vi "AxesPositions.vi"(0 "System no.":i32=1 min=1 step=1, 5 "error in":errorcluster) -> (19 "error out":errorcluster)   [LabVIEW 2014]
doc: "This VI allows to save position information to a text file. Also the position information from a text file can be opened again.\nPressing on the \"Stop Motion (F10)\" or the F10 key will send a \"#24\" command to the controller to stop the motion of every axis.\nThis VI opens modal so that the communication, especially the STOP command, is not disturbed by any other processes."
uses:
  C:/ProgramData/PI/LabVIEW/Low Level/General command.llb/Global2 (Array).vi
panel:
  in  "Move to target":bool[](array[boolean])
  in  "Save to file":bool
  in  "Load from file":bool
  in  "Current to Target":bool
  in  "Target Position":dbl[](array[numeric]) format="%.6f"
  out "Conn. axes":string[](array[string])
  out "Current Position":dbl[](array[numeric]) format="%.6f"
  in  "Stop Motion":bool
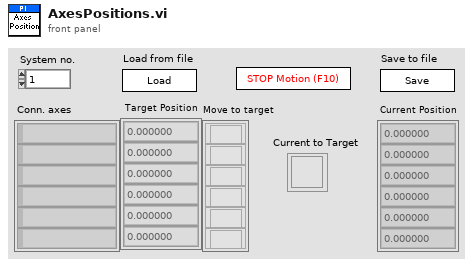
[diagram p1: front panel]
types:
  T1 = enum16{"open", "replace", "create", "open or create", "replace or create", "replace or create with confirmation"}
  T2 = typedef "Controller names.ctl" = enum16{"None", "Analog", "C-702", "C-413", "C-414", "C-843", "C-843.PM", "C-844", "C-848", "C-865", "C-866", "C-867", "C-877", "C-880", "C-884", "C-885", "C-886", "C-887", "C-891", "E-135", "E-516", "E-517", "E-518", "E-709", "E-710", "E-712", "E-725", "E-727", "E-753", "E-754", "E-755", "E-761", "E-816", "E-861", "E-870", "E-871", "E-872", "E-873", "E-874", "F-206", "HydraPollux", "M-840", "M-850", "M-8X0", "Mercury", "Mercury_GCS", "PI_GCS2"}
  T3 = cluster{"Conn. axes":string[], "Controller name":T2}[]
  T4 = cluster{"Conn. axes":string[], "Controller name":T2}
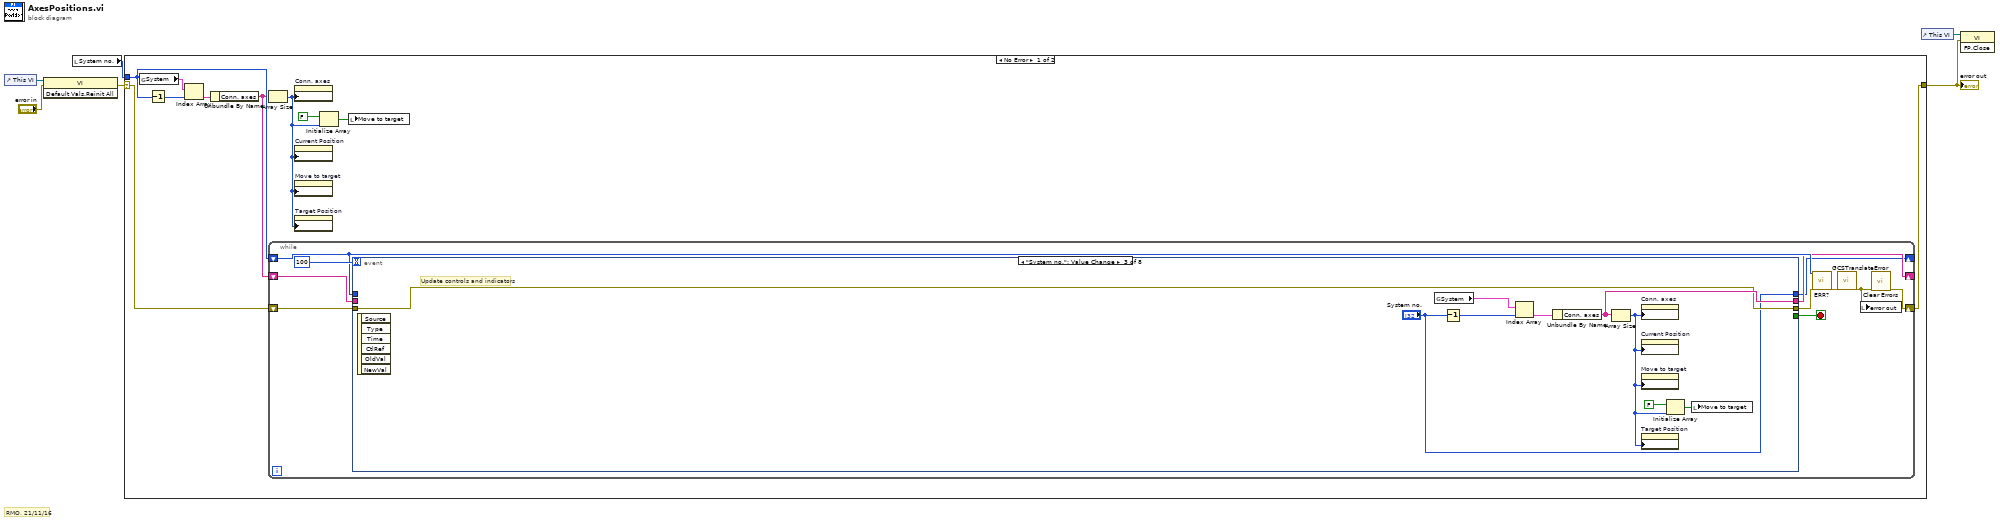
[diagram p0: block diagram]
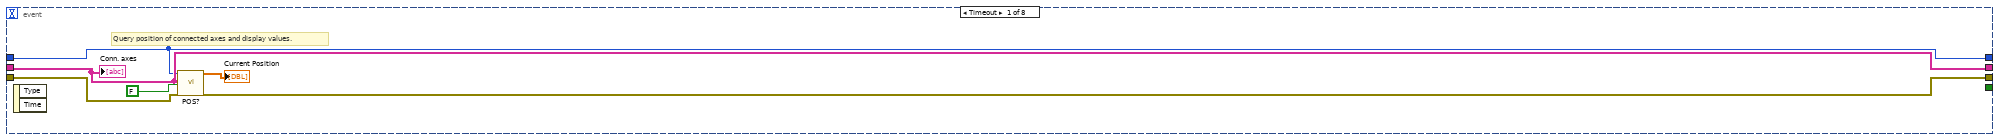
[diagram p2: hidden frame]
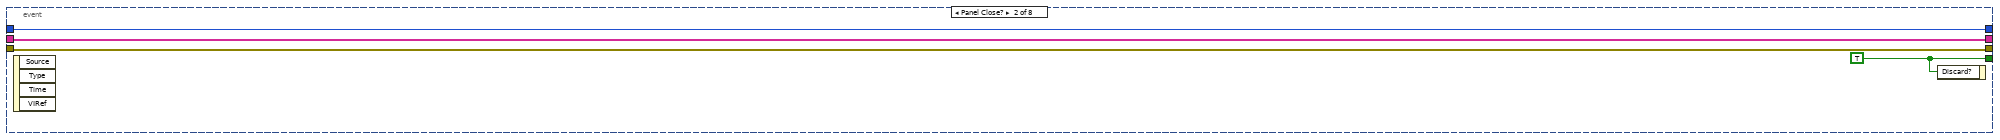
[diagram p3: hidden frame]
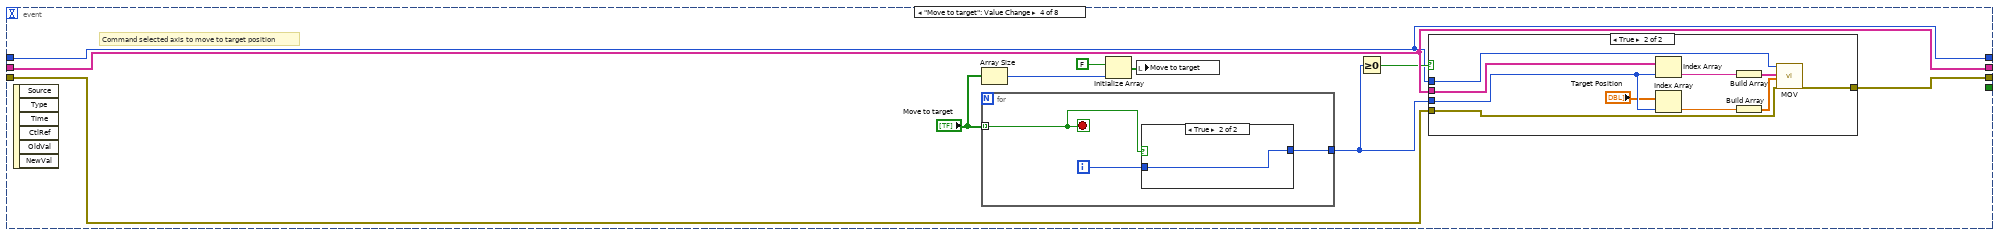
[diagram p4: hidden frame]
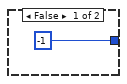
[diagram p6: hidden frame]
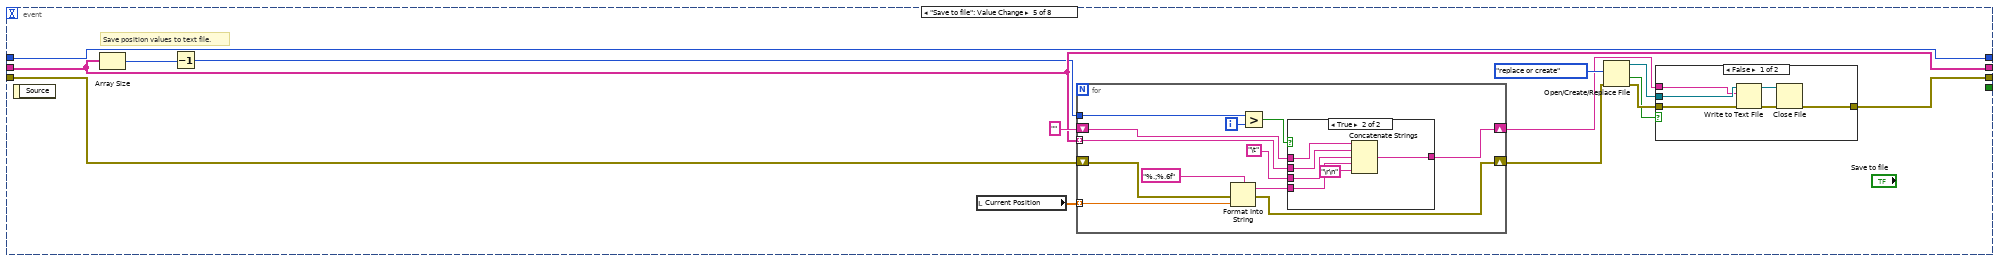
[diagram p7: hidden frame]
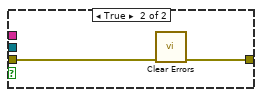
[diagram p8: hidden frame]
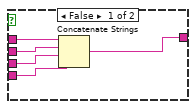
[diagram p9: hidden frame]
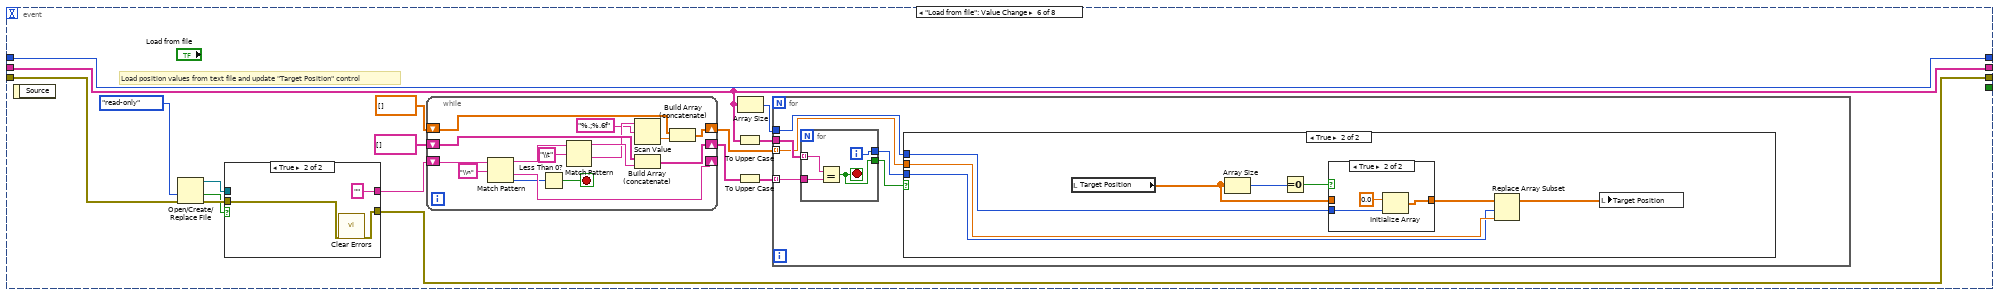
[diagram p10: hidden frame]
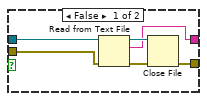
[diagram p11: hidden frame]
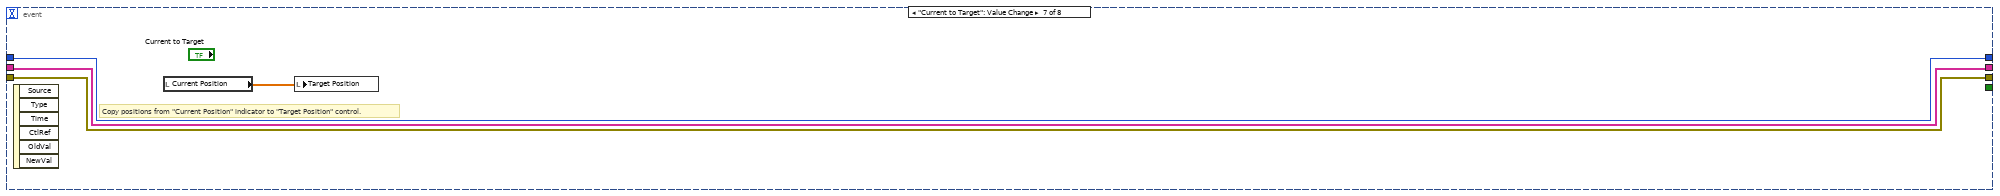
[diagram p14: hidden frame]
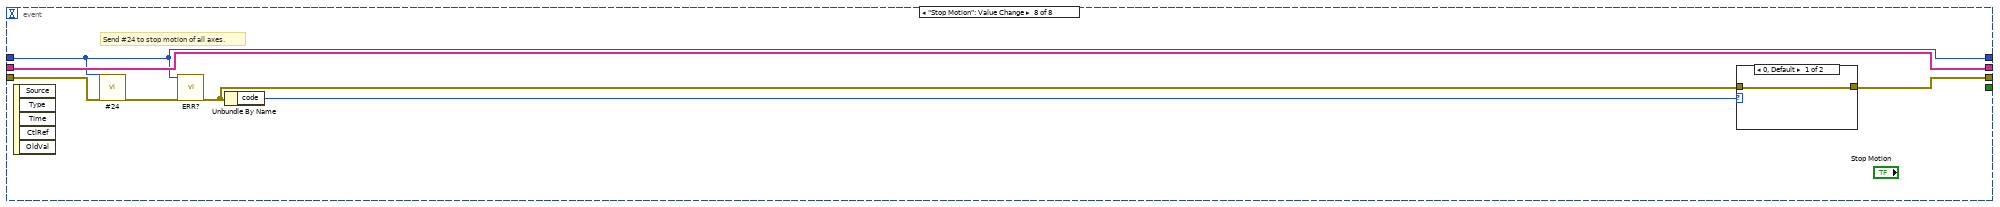
[diagram p15: hidden frame]
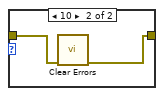
[diagram p16: hidden frame]
diagram:
  # "RMO, 21/11/16"
  n1 = control-ref of="This VI"() -> (w5:refnum<vi>)
  n2 = invoke class="VI" method="Default Vals.Reinit All"(reference=w5, error in="error in") -> (error out=w3:errorcluster)  [unwired: 1 in, 2 out]
  n3 = local read "System no."() -> (w1:i32)
  n4 = case shown="No Error" w3 {
    selector: w3 -> [w11 w194]
    tunnel: [w13 w194] -> w6
    tunnel: w1 -> [w12 _]
    frame No Error {
      n5 = global read "Global2 (Array).vi" "System"() -> (w16:T3)
      n6 = Decrement(x=w12) -> (x-1=w15:i32)
      n7 = Index Array(array=w16, index=w15) -> (element=w14:T4)
      n8 = Unbundle By Name(w14) -> ("Conn. axes"=w10:string[])
      n9 = Array Size(array=w10) -> (size(s)=w7:i32)
      n10 = while {
        shift-right: [w20] -> w13
        shift-left: w11 -> [w26]
        shift-right: [w18] -> _
        shift-left: w10 -> [w27]
        shift-right: [w17] -> _
        shift-left: w12 -> [w21]
        stop <- w25 stop-if-true
        n11 = event shown="[2] \"System no.\": Value Change" {
          selector: _ -> [_ _ _ _ _ _ _ _]
          dyn-events: _ -> [_ _ _ _ _ _ _ _]
          timeout: 100 -> [_ _ _ _ _ _ _ _]
          tunnel: w27 -> [w29 w36 _ w52 w84 w120 w181 w190]
          tunnel: w26 -> [w33 w35 w39 w49 w81 w133 w183 w189]
          tunnel: [w32 w35 w39 w48 w75 w122 w183 w185] -> w23
          tunnel: [_ w37 _ _ _ _ _ _] -> w25
          tunnel: w21 -> [w28 w34 _ w47 w73 w118 w180 w184]
          tunnel: [w29 w36 w43 w52 w84 w120 w181 w190] -> w18
          tunnel: [w28 w34 "System no." w47 w73 w118 w180 w184] -> w17
          event Timeout {
            # "Query position of connected axes and display values."
            n12 = event-data() -> ()  [unwired: 3 out]
            n13 = call "POS?.vi"("System no."=w28, "Axes to query"=w29, "All axes?"=FALSE, "error in"=w33) -> ("Position"=→"Current Position":dbl[], "error out"=w32:errorcluster)  [unwired: 1 in, 13 out]
            "Conn. axes" <- w29
          }
          event Panel Close? {
            w37 = TRUE
            n14 = event-data() -> ()  [unwired: 5 out]
            n15 = event-data("Discard?"=w37) -> ()  [unwired: 1 in, 1 out]
          }
          event "System no.": Value Change {
            # "Update controls and indicators"
            n16 = event-data() -> ()  [unwired: 7 out]
            n17 = global read "Global2 (Array).vi" "System"() -> (w44:T3)
            n18 = Decrement(x="System no.") -> (x-1=w45:i32)
            n19 = Index Array(array=w44, index=w45) -> (element=w46:T4)
            n20 = Unbundle By Name(w46) -> ("Conn. axes"=w43:string[])
            n21 = Array Size(array=w43) -> (size(s)=w40:i32)
            n22 = property on="Conn. axes" class="Arr (strict)"("Number of Rows"=w40) -> ()  [unwired: 2 in, 2 out]
            n23 = property on="Current Position" class="Arr (strict)"("Number of Rows"=w40) -> ()  [unwired: 2 in, 2 out]
            n24 = property on="Move to target" class="Arr"("Number of Rows"=w40) -> ()  [unwired: 2 in, 2 out]
            n25 = property on="Target Position" class="Arr (strict)"("Number of Rows"=w40) -> ()  [unwired: 2 in, 2 out]
            n26 = Initialize Array(FALSE, w40) -> (w42:bool[])
            n27 = local write "Move to target"(w42) -> ()
          }
          event "Move to target": Value Change {
            # "Command selected axis to move to target position"
            n28 = event-data() -> ()  [unwired: 7 out]
            n29 = Array Size(array="Move to target") -> (size(s)=w55:i32)
            n30 = for {
              tunnel: "Move to target" -> [w70] mode=indexing
              tunnel: [w68] -> w50
              i -> [w69]
              stop <- w70 stop-if-true
              n31 = case shown="True" w70 {
                tunnel: w69 -> [_ w72]
                tunnel: [-1 w72] -> w68
                frame False {
                }
                frame True {
                }
              }
            }
            n32 = Initialize Array(FALSE, w55) -> (w54:bool[])
            n33 = local write "Move to target"(w54) -> ()
            n34 = Greater Or Equal To 0?(x=w50) -> (x >= 0?=w51:bool)
            n35 = case shown="True" w51 {
              tunnel: w52 -> [_ w67]
              tunnel: w50 -> [_ w66]
              tunnel: w47 -> [_ w62]
              tunnel: w49 -> [w57 w64]
              tunnel: [w57 w63] -> w48
              frame False {
              }
              frame True {
                n36 = Index Array(array=w67, index=w66) -> (element=w61:string)
                n37 = Index Array(array="Target Position", index=w66) -> (element=w60:dbl)
                n38 = Build Array(w61) -> (w59:string[])
                n39 = Build Array(w60) -> (w58:dbl[])
                n40 = call "MOV.vi"("System no."=w62, "Axes to move"=w59, "Position values"=w58, "error in"=w64) -> ("error out"=w63:errorcluster)  [unwired: 1 in, 14 out]
              }
            }
          }
          event "Save to file": Value Change {
            # "Save position values to text file."
            n41 = event-data() -> ()  [unwired: 2 out]
            n42 = Array Size(array=w84) -> (size(s)=w83:i32)
            n43 = Decrement(x=w83) -> (x-1=w82:i32)
            n44 = local read "Current Position"() -> (w85:dbl[])
            n45 = for {
              shift-right: [w97] -> w76
              shift-left: "" -> [w104]
              tunnel: w84 -> [w103] mode=indexing
              tunnel: w85 -> [w105] mode=indexing
              tunnel: w82 -> [w100]
              shift-right: [w95] -> w80
              shift-left: w81 -> [w96]
              i -> [w99]
              n46 = Format Into String(format string="%.;%.6f", error in=w96, w105) -> (resulting string=w101:string, error out=w95:errorcluster)  [unwired: 1 in]
              n47 = Greater?(x=w100, y=w99) -> (0:w98:bool)
              n48 = case shown="True" w98 {
                tunnel: w104 -> [w111 w117]
                tunnel: w103 -> [w110 w116]
                tunnel: "\t" -> [w109 w115]
                tunnel: w101 -> [w108 w114]
                tunnel: [w107 w112] -> w97
                frame False {
                  n49 = Concatenate Strings(w111, w110, w109, w108) -> (w107:string)
                }
                frame True {
                  n50 = Concatenate Strings(w117, w116, w115, w114, "\r\n") -> (w112:string)
                }
              }
            }
            n51 = Open/Create/Replace File(error in=w80, operation (0:open)=T1."replace or create") -> (refnum out=w77:refnum<file>, cancelled=w74:bool, error out=w78:errorcluster)  [unwired: 4 out]
            n52 = case shown="False" w74 {
              tunnel: w78 -> [w92 w94]
              tunnel: w77 -> [w91 _]
              tunnel: w76 -> [w90 _]
              tunnel: [w87 w93] -> w75
              frame False {
                n53 = Write to Text File(file (use dialog)=w91, text=w90, error in=w92) -> (refnum out=w88:refnum<file>, error out=w89:errorcluster)  [unwired: 2 out]
                n54 = Close File(refnum=w88, error in=w89) -> (error out=w87:errorcluster)  [unwired: 1 out]
              }
              frame True {
                n55 = call <vilib>:"Clear Errors.vi"("error in (no error)"=w94) -> ("error out"=w93:errorcluster)  [unwired: 1 in, 5 out]
              }
            }
          }
          event "Load from file": Value Change {
            # "Load position values from text file and update \"Target Position\" control"
            n56 = event-data() -> ()  [unwired: 2 out]
            n57 = Open/Create/Replace File(error in=w133, access (0:read/write)=enum16{"read/write", "read-only", "write-only"}."read-only") -> (refnum out=w130:refnum<file>, cancelled=w121:bool, error out=w131:errorcluster)  [unwired: 4 out]
            n58 = case shown="True" w121 {
              tunnel: w131 -> [w139 w141]
              tunnel: w130 -> [w138 _]
              tunnel: [w135 ""] -> w128
              tunnel: [w134 w140] -> w122
              frame False {
                n59 = Read from Text File(file (use dialog)=w138, error in=w139) -> (refnum out=w136:refnum<file>, text=w135:string, error out=w137:errorcluster)  [unwired: 3 out]
                n60 = Close File(refnum=w136, error in=w137) -> (error out=w134:errorcluster)  [unwired: 1 out]
              }
              frame True {
                n61 = call <vilib>:"Clear Errors.vi"("error in (no error)"=w141) -> ("error out"=w140:errorcluster)  [unwired: 1 in, 5 out]
              }
            }
            n62 = while {
              shift-right: [w175] -> w127
              shift-left: string[] [] -> [w177]
              shift-right: [w176] -> _
              shift-left: w128 -> [w179]
              shift-right: [w168] -> w123
              shift-left: dbl[] [] -> [w169]
              stop <- w173 stop-if-true
              n63 = Match Pattern(string=w179, regular expression="\\n") -> (before substring=w171:string, after substring=w176:string, offset past match=w174:i32)  [unwired: 2 out]
              n64 = Less Than 0?(x=w174) -> (x < 0?=w173:bool)
              n65 = Match Pattern(string=w171, regular expression="\\t") -> (before substring=w170:string, after substring=w167:string)  [unwired: 3 out]
              n66 = Scan Value(string=w167, format string="%.;%.6f") -> (value=w165:dbl)  [unwired: 2 out]
              n67 = Build Array (concatenate)(w177, w170) -> (w175:string[])
              n68 = Build Array (concatenate)(w169, w165) -> (w168:dbl[])
            }
            n69 = To Upper Case(1:w120) -> (0:w124:string[])
            n70 = To Upper Case(1:w127) -> (0:w125:string[])
            n71 = Array Size(array=w120) -> (size(s)=w119:i32)
            n72 = for {
              tunnel: w125 -> [w147] mode=indexing
              tunnel: w124 -> [w148]
              tunnel: w123 -> [w146] mode=indexing
              tunnel: w119 -> [w143]
              n73 = for {
                tunnel: w148 -> [w164] mode=indexing
                tunnel: w147 -> [w163]
                tunnel: [w162] -> w145
                tunnel: [w161] -> w144
                i -> [w161]
                stop <- w162 stop-if-true
                n74 = Equal?(x=w164, y=w163) -> (x = y?=w162:bool)
              }
              n75 = case shown="True" w145 {
                tunnel: w146 -> [_ w156]
                tunnel: w144 -> [_ w155]
                tunnel: w143 -> [_ w150]
                frame False {
                }
                frame True {
                  n76 = local read "Target Position"() -> (w151:dbl[])
                  n77 = Array Size(array=w151) -> (size(s)=w153:i32)
                  n78 = Equal To 0?(x=w153) -> (x = 0?=w152:bool)
                  n79 = case shown="True" w152 {
                    tunnel: w151 -> [w157 _]
                    tunnel: w150 -> [_ w159]
                    tunnel: [w157 w158] -> w149
                    frame False {
                    }
                    frame True {
                      n80 = Initialize Array(0.0 ("element"), w159) -> (w158:dbl[])
                    }
                  }
                  n81 = Replace Array Subset(array=w149, new element=w156, index=w155) -> (w154:dbl[])
                  n82 = local write "Target Position"(w154) -> ()
                }
              }
            }
          }
          event "Current to Target": Value Change {
            # "Copy positions from \"Current Position\" indicator to \"Target Position\" control."
            n83 = event-data() -> ()  [unwired: 7 out]
            n84 = local read "Current Position"() -> (w182:dbl[])
            n85 = local write "Target Position"(w182) -> ()
          }
          event "Stop Motion": Value Change {
            # "Send #24 to stop motion of all axes."
            n86 = event-data() -> ()  [unwired: 6 out]
            n87 = call "#24.vi"("System no."=w184, "error in"=w189) -> ("error out"=w188:errorcluster)  [unwired: 17 out]
            n88 = call "ERR?.vi"("System no."=w184, "error in"=w188) -> ("error out"=w186:errorcluster)  [unwired: 17 out]
            n89 = Unbundle By Name(w186) -> ("code"=w187:i32)
            n90 = case shown="0, Default" w187 {
              tunnel: w186 -> [w191 w193]
              tunnel: [w191 w192] -> w185
              frame 0, Default {
              }
              frame 10 {
                n91 = call <vilib>:"Clear Errors.vi"("error in (no error)"=w193) -> ("error out"=w192:errorcluster)  [unwired: 1 in, 5 out]
              }
            }
          }
        }
        n92 = call "ERR?.vi"("System no."=w21, "error in"=w23) -> ("error out"=w22:errorcluster)  [unwired: 17 out]
        n93 = call "GCSTranslateError.vi"("error in"=w22) -> ("error out"=w19:errorcluster)  [unwired: 18 out]
        n94 = local write "error out"(w19) -> ()
        n95 = call <vilib>:"Clear Errors.vi"("error in (no error)"=w19) -> ("error out"=w20:errorcluster)  [unwired: 1 in, 5 out]
      }
      n96 = property on="Conn. axes" class="Arr (strict)"("Number of Rows"=w7) -> ()  [unwired: 2 in, 2 out]
      n97 = property on="Current Position" class="Arr (strict)"("Number of Rows"=w7) -> ()  [unwired: 2 in, 2 out]
      n98 = property on="Move to target" class="Arr"("Number of Rows"=w7) -> ()  [unwired: 2 in, 2 out]
      n99 = property on="Target Position" class="Arr (strict)"("Number of Rows"=w7) -> ()  [unwired: 2 in, 2 out]
      n100 = Initialize Array(FALSE, w7) -> (w8:bool[])
      n101 = local write "Move to target"(w8) -> ()
    }
    frame Error {
    }
  }
  "error out" <- w6
  n102 = control-ref of="This VI"() -> (w2:refnum<vi>)
  n103 = invoke class="VI" method="FP.Close"(reference=w2, error in=w6) -> ()  [unwired: 1 in, 3 out]
